vi "Enable Output.vi"(8 "error in (no error)":errorcluster, 10 "Enable Output (T: Enable)":bool=TRUE, 11 "VISA resource name":refnum<visa-resource-name>) -> (0 "error out":errorcluster, 3 "VISA resource name out":refnum<visa-resource-name>)   [LabVIEW 2020, in "Keithley 24XX.lvlib"]
doc: "Enables the source to output the assigned voltage or current to the device under test. The output must be enabled to make measurements, regardless of the output settings."
uses:
  <instrlib>/Keithley 24XX/Keithley 24XX.lvlib
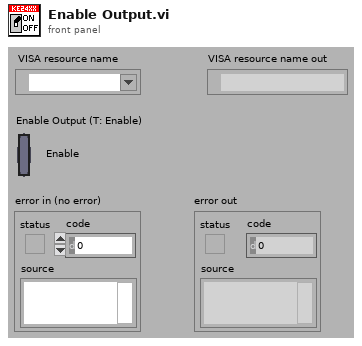
[diagram p1: front panel]
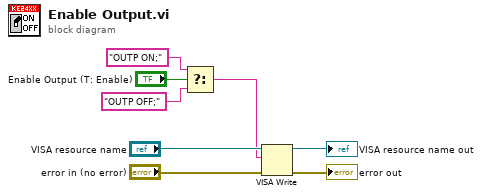
[diagram p0: block diagram]
diagram:
  n1 = Select(t="OUTP ON;", s="Enable Output (T: Enable)", f="OUTP OFF;") -> (s? t:f=w1:string)
  n2 = VISA Write(VISA resource name="VISA resource name", write buffer=w1, error in (no error)="error in (no error)") -> (VISA resource name out=→"VISA resource name out":refnum<visa-resource-name>, error out=→"error out":errorcluster)  [unwired: 1 out]
